vi "SemiManualScript.vi"   [LabVIEW 2024, in "CustomActions.lvlib"]
uses:
  CustomActions.lvlib
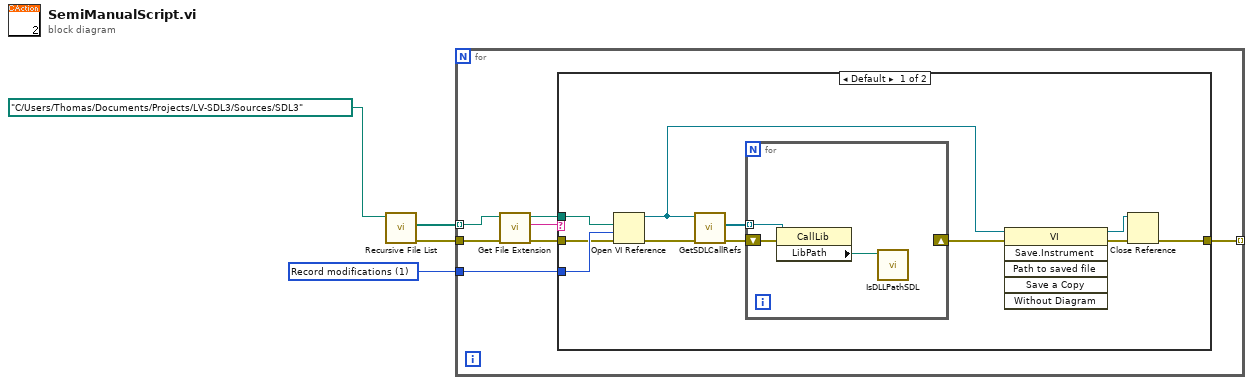
[diagram p0: block diagram]
diagram:
  w2 = 1 items=["Record modifications"=1, "Open templates for editing"=2, "Prompt user to save"=4, "Prepare for reentrant run"=8, "Prompt to find missing subVIs"=16, "Hide loading dialog box"=32, "Enable simultaneous calls"=64, "Prepare to call and forget"=128, "Simultaneous call and forget"=192, "Prepare to call and collect"=256, "Simultaneous call and collect"=320]
  n1 = call <vilib>:"Recursive File List.vi"("Folder Path"=path "C:/Users/Thomas/Documents/Projects/LV-SDL3/Sources/SDL3") -> ("error out"=w1:errorcluster, "All Files in Dir"=w3:path[])  [unwired: 6 in, 3 out]
  n2 = for {
    tunnel: w3 -> [w11] mode=indexing
    tunnel: w2 -> [w8]
    tunnel: [w7] -> _ mode=indexing
    tunnel: w1 -> [w6]
    n3 = call <vilib>:"Get File Extension.vi"("error in (no error)"=w6, "file"=w11) -> ("error out"=w5:errorcluster, "lowercase file extension"=w10:string, "dup file"=w9:path)  [unwired: 5 in, 2 out]
    n4 = case shown="Default" w10 {
      tunnel: w9 -> [w22 _]
      tunnel: w8 -> [w21 _]
      tunnel: [w14 w26] -> w7
      tunnel: w5 -> [w13 w26]
      frame Default {
        n5 = Open VI Reference(vi path=w22, options=w21, error in (no error)=w13) -> (vi reference=w18:refnum<vi>, error out=w20:errorcluster)  [unwired: 3 in]
        n6 = call "GetSDLCallRefs.vi"("error in (no error)"=w20, "VI Refnum"=w18) -> ("error out"=w16:errorcluster, "VI SDL Call Nodes"=w12:refnum<vi>[])  [unwired: 8 in]
        n7 = for {
          shift-right: [_] -> w15
          shift-left: w16 -> [w24]
          tunnel: w12 -> [w25] mode=indexing
          n8 = property class="CallLib"(reference=w25, error in=w24) -> ("LibPath"=w23:path)  [unwired: 2 out]
          n9 = call "IsDLLPathSDL.vi"("DLL Path"=w23) -> ()  [unwired: 7 in, 4 out]
        }
        n10 = invoke class="VI" method="Save.Instrument"(reference=w18, error in=w15) -> (reference out=w17:refnum<vi>, error out=w19:errorcluster)  [unwired: 4 in, 4 out]
        n11 = Close Reference(reference=w17, error in (no error)=w19) -> (error out=w14:errorcluster)
      }
      frame "vi", "vim" {
      }
    }
  }
